vi "Scripting_GetStateMachineReferences.vi"() -> ()   [LabVIEW 2020]
panel:
  in  "Path":path=path "C:/Documents and Settings/MikaelH/My Documents/LabView/StateMachine-JKI/StateMachine1.vi"
  out "ErrorOut":errorcluster
  in  "ErrorIn":errorcluster
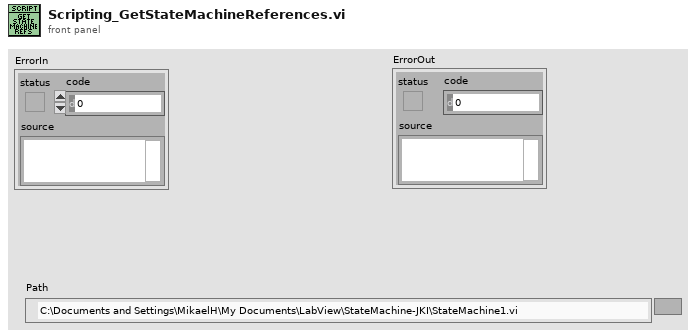
[diagram p1: front panel]
types:
  T1 = cluster{"StateMachineCaseSelector":refnum<vi>, "StateWhileLoopDiagram":refnum<vi>, "OutSideWhileLoopDiagram":refnum<vi>, "Selector.Outside Terminal":refnum<vi>, "vi reference":refnum<vi>}
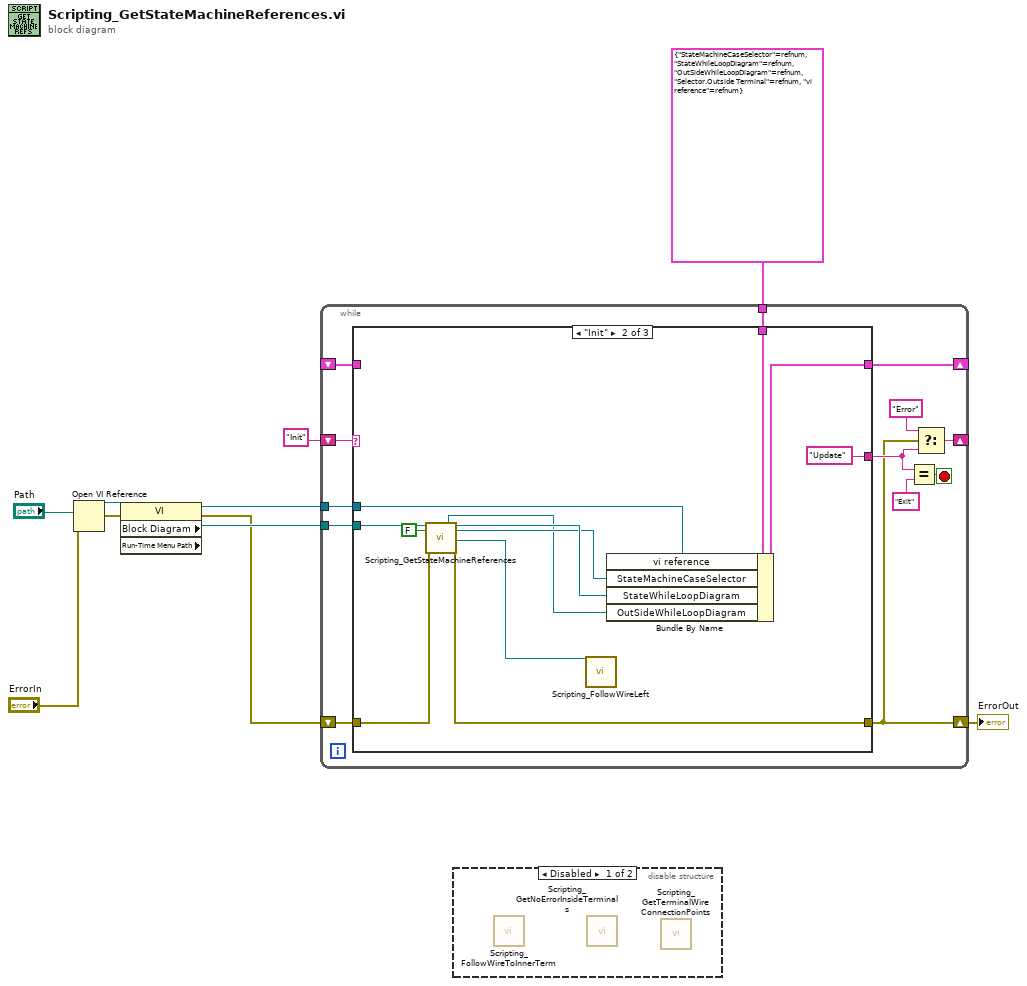
[diagram p0: block diagram]
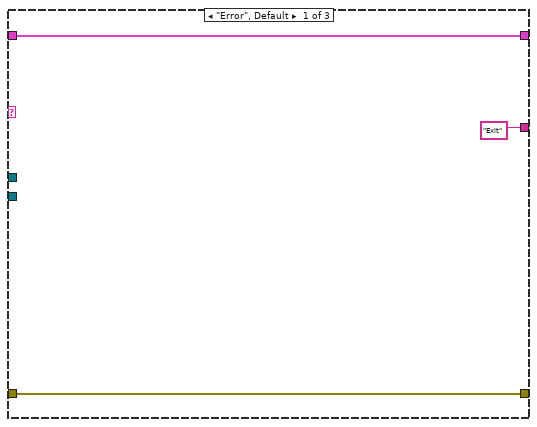
[diagram p3: hidden frame]
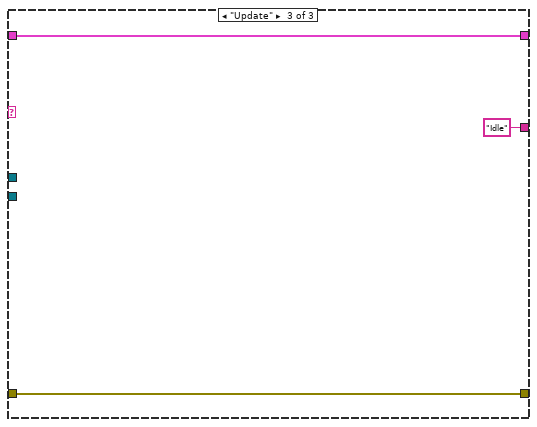
[diagram p4: hidden frame]
diagram:
  n1 = Open VI Reference(vi path="Path", error in (no error)="ErrorIn") -> (vi reference=w8:refnum<vi>, error out=w5:errorcluster)  [unwired: 1 in, 3 out]
  n2 = property class="VI" props=["Block Diagram", "Run-Time Menu Path"](reference=w8, error in=w5) -> (reference out=w2:refnum<vi>, error out=w4:errorcluster, "Block Diagram"=w6:refnum<vi>)  [unwired: 1 out]
  n3 = while {
    shift-right: [w16] -> w9
    shift-left: w4 -> [w23]
    shift-right: [w21] -> _
    shift-left: "Init" -> [w22]
    shift-right: [w15] -> _
    shift-left: _ -> [w14]
    tunnel: w6 -> [w13]
    tunnel: w2 -> [w12]
    tunnel: T1 {"StateMachineCaseSelector"=refnum, "StateWhileLoopDiagram"=refnum, "OutSideWhileLoopDiagram"=refnum, "Selector.Outside Terminal"=refnum, "vi reference"=refnum} -> [w11]
    stop <- w20 stop-if-true
    n4 = case shown="\"Init\"" w22 {
      tunnel: w23 -> [w26 w32 w39]
      tunnel: [w26 w31 w39] -> w16
      tunnel: ["Exit" "Update" "Idle"] -> w17
      tunnel: [w24 w37 w40] -> w15
      tunnel: w14 -> [w24 _ w40]
      tunnel: w13 -> [_ w36 _]
      tunnel: w12 -> [_ w28 _]
      tunnel: w11 -> [_ w29 _]
      frame "Error", Default {
      }
      frame "Init" {
        n5 = call "Scripting_GetStateMachineReferences.vi"("Diagram"=w36, "WhileLoop(False)"=FALSE, "error in (no error)"=w32) -> ("OutSideWhileLoopDiagram"=w33:refnum<vi>, "StateMachine-WhileLoopDiagram"=w35:refnum<vi>, "StateMachine-CaseSelector"=w34:refnum<vi>, "Selector.Outside Terminal"=w30:refnum<vi>, "error out"=w31:errorcluster)  [unwired: 11 in, 1 out]
        n6 = call "Scripting_FollowWireLeft.vi"("Term Refnum"=w30) -> ()  [unwired: 15 in, 4 out]
        n7 = Bundle By Name(cluster=w29, "vi reference"=w28, "StateMachineCaseSelector"=w34, "StateWhileLoopDiagram"=w35, "OutSideWhileLoopDiagram"=w33) -> (w37:T1)
      }
      frame "Update" {
      }
    }
    n8 = Equal?(x=w17, y="Exit") -> (x = y?=w20:bool)
    n9 = Select(t="Error", s=w16, f=w17) -> (s? t:f=w21:string)
  }
  "ErrorOut" <- w9
  n10 = disable-structure shown="Disabled" {
    frame Disabled {
      n11 = call "Scripting_FollowWireToInnerTerm.vi"() -> ()  [unwired: 18 in, 2 out]
      n12 = call "Scripting_GetNoErrorInsideTerminals.vi"() -> ()  [unwired: 13 in, 7 out]
      n13 = call "Scripting_GetTerminalWireConnectionPoints.vi"() -> ()  [unwired: 11 in, 9 out]
    }
    frame Enabled {
    }
  }
